vi "Restart Unit.vi"(8 "error in (no error)":errorcluster, 10 "New IP (empty = original)":string, 11 "ENET in":refnum<class "ENET_BS120x.lvclass">) -> (0 "error out":errorcluster, 3 "ENET out":refnum<class "ENET_BS120x.lvclass">)   [LabVIEW 2021, in "BS120x Driver.lvlib" / "ENET_BS120x.lvclass"]
uses:
  ENET_BS120x.lvclass
  ENET_BS120x.lvclass/ENET_BS120x.ctl
panel:
  out "Num Tries":i32
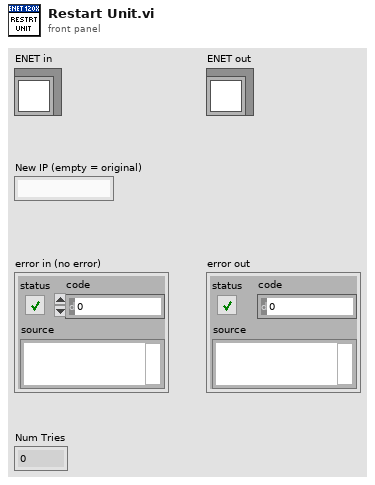
[diagram p1: front panel]
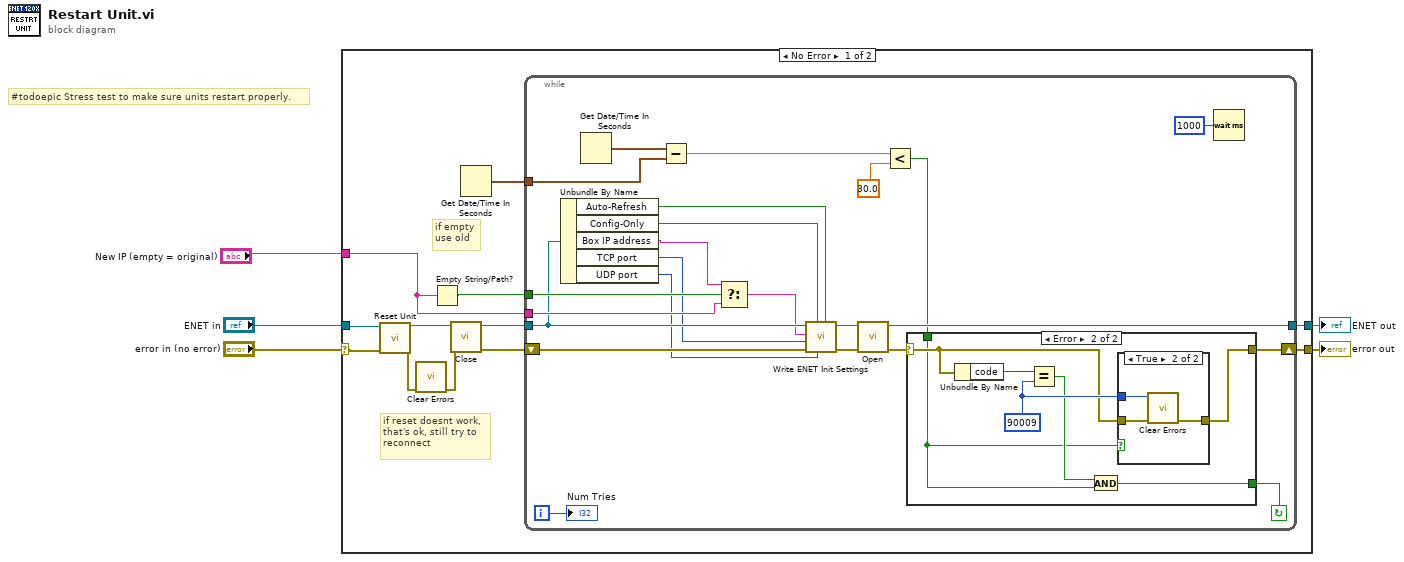
[diagram p0: block diagram]
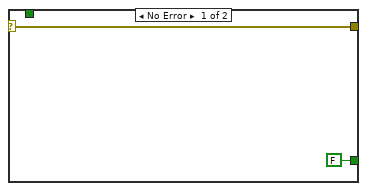
[diagram p2: hidden frame]
diagram:
  # "#todoepic Stress test to make sure units restart properly."
  n1 = case shown="No Error" "error in (no error)" {
    selector: "error in (no error)" -> [w8 w54]
    tunnel: [w17 w54] -> w5
    tunnel: [w16 w55] -> w4
    tunnel: "ENET in" -> [w10 w55]
    tunnel: "New IP (empty = original)" -> [w11 _]
    frame No Error {
      # "if reset doesnt work,\nthat's ok, still try to\nreconnect"
      # "if empty\nuse old"
      n2 = call-dynamic "Reset Unit.vi"("error in (no error)"=w8, "Ethernet in"=w10) -> ("error out"=w7:errorcluster, "Ethernet out"=w9:refnum<class "ENET_BS120x.lvclass">)  [unwired: 8 in]
      n3 = call <vilib>:"Clear Errors.vi"("error in (no error)"=w7) -> ("error out"=w6:errorcluster)  [unwired: 5 in, 1 out]
      n4 = Empty String/Path?(string/path=w11) -> (empty?=w12:bool)
      n5 = call-dynamic "Close.vi"("error in (no error)"=w6, "ENET in"=w9) -> ("error out"=w13:errorcluster, "ENET out"=w14:refnum<class "ENET_BS120x.lvclass">)  [unwired: 8 in]
      n6 = Get Date/Time In Seconds() -> (seconds since 1Jan1904=w15:timestamp)
      n7 = while {
        tunnel: [w40] -> w16
        tunnel: w14 -> [w24]
        shift-right: [w39] -> w17
        shift-left: w13 -> [w23]
        tunnel: w15 -> [w37]
        tunnel: w12 -> [w29]
        tunnel: w11 -> [w27]
        i -> [w30]
        stop <- w32 continue-if-true
        n8 = Unbundle By Name(w24) -> ("Auto-Refresh"=w22:bool, "Config-Only"=w21:bool, "Box IP address"=w28:string, "TCP port"=w19:u16, "UDP port"=w18:u16)
        n9 = Get Date/Time In Seconds() -> (seconds since 1Jan1904=w38:timestamp)
        n10 = Subtract(x=w38, y=w37) -> (x-y=w36:dbl)
        n11 = Select(t=w28, s=w29, f=w27) -> (s? t:f=w20:string)
        n12 = call-dynamic "Write ENET Init Settings.vi"("Auto-Refresh (T)"=w22, "UDP port"=w18, "Connect for Config Only? (F)"=w21, "error in (no error)"=w23, "TCP port"=w19, "Box IP address"=w20, "Ethernet_BS1201 in"=w24) -> ("error out"=w25:errorcluster, "Ethernet_BS1201 out"=w26:refnum<class "ENET_BS120x.lvclass">)  [unwired: 3 in]
        n13 = call-dynamic "Open.vi"("error in (no error)"=w25, "ENET In"=w26) -> ("error out"=w34:errorcluster, "ENET out"=w40:refnum<class "ENET_BS120x.lvclass">)  [unwired: 8 in]
        n14 = Less?(x=w36, y=30.0) -> (x < y?=w33:bool)
        n15 = case shown="Error" w34 {
          selector: w34 -> [w42 w46]
          tunnel: [w42 w48] -> w39
          tunnel: w33 -> [_ w43]
          tunnel: [FALSE w44] -> w32
          frame No Error {
          }
          frame Error {
            w47 = 90009 ("y")
            n16 = Unbundle By Name(w46) -> ("code"=w49:i32)
            n17 = Equal?(x=w49, y=w47) -> (x = y?=w45:bool)
            n18 = And(x=w45, y=w43) -> (x .and. y?=w44:bool)
            n19 = case shown="True" w43 {
              tunnel: [w50 w53] -> w48
              tunnel: w47 -> [_ w52]
              tunnel: w46 -> [w50 w51]
              frame False {
              }
              frame True {
                n20 = call <vilib>:"Clear Errors.vi"("error in (no error)"=w51, "specific error code to clear (0: all)"=w52) -> ("error out"=w53:errorcluster)  [unwired: 4 in, 1 out]
              }
            }
          }
        }
        n21 = Wait (ms)(milliseconds to wait=u32 1000) -> ()  [unwired: 1 out]
        "Num Tries" <- w30
      }
    }
    frame Error {
    }
  }
  "error out" <- w5
  "ENET out" <- w4
